vi "LJUD_Close.vi"(8 "error in":errorcluster) -> (0 "error out":errorcluster)   [LabVIEW 2020]
uses:
  Library/Frameworks/LabJackM.framework
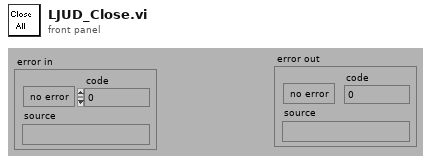
[diagram p1: front panel]
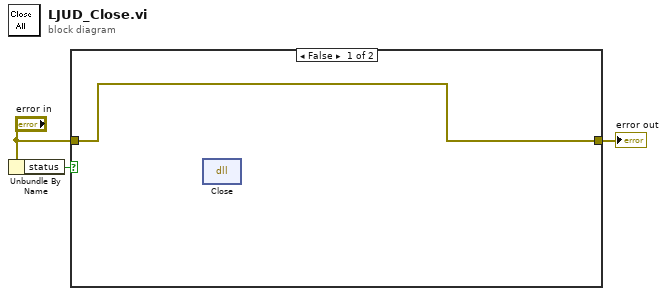
[diagram p0: block diagram]
diagram:
  n1 = Unbundle By Name("error in") -> ("status"=w2:bool)
  n2 = case shown="False" w2 {
    tunnel: [w4 w5] -> w3
    tunnel: "error in" -> [w4 w5]
    frame False {
      n3 = dll-call lib="Library/Frameworks/LabJackM.framework" fn="Close"() -> ()  [unwired: 4 in, 2 out]
    }
    frame True {
    }
  }
  "error out" <- w3
